vi "Get SMO Port.vi"(8 "error in (no error)":errorcluster, 11 "Inst.TCInstrument in":refnum<class "Inst.TC.lvclass">) -> (0 "error out":errorcluster, 2 "Port":u16, 3 "Inst.TCInstrument out":refnum<class "Inst.TC.lvclass">)   [LabVIEW 2019, in "Inst.TC.lvclass"]
uses:
  Inst.TC.lvclass
  <userlib>/LevyLab/Instrument Framework/Instrument Types/VSource/Instrument.VSource.lvclass
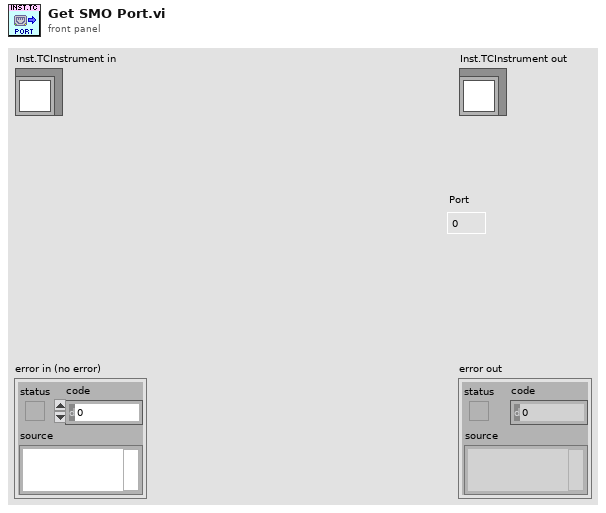
[diagram p1: front panel]
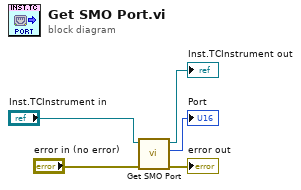
[diagram p0: block diagram]
diagram:
  n1 = call-parent "Get SMO Port.vi"("error in (no error)"="error in (no error)", "Instrument in"="Inst.TCInstrument in") -> ("error out"=→"error out":errorcluster, "Port"=→"Port":u16, "Instrument out"=→"Inst.TCInstrument out":refnum<class "Inst.TC.lvclass">)  [unwired: 7 in]
